vi "Test Complete.vi"(8 "Vehicle":string, 9 "SMS Recipients":u32, 10 "Send SMS":bool, 11 "File Name":string) -> ()   [LabVIEW 2014]
panel:
  out "Boolean array":bool[](array[boolean])
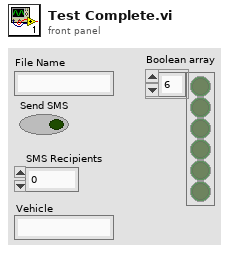
[diagram p1: front panel]
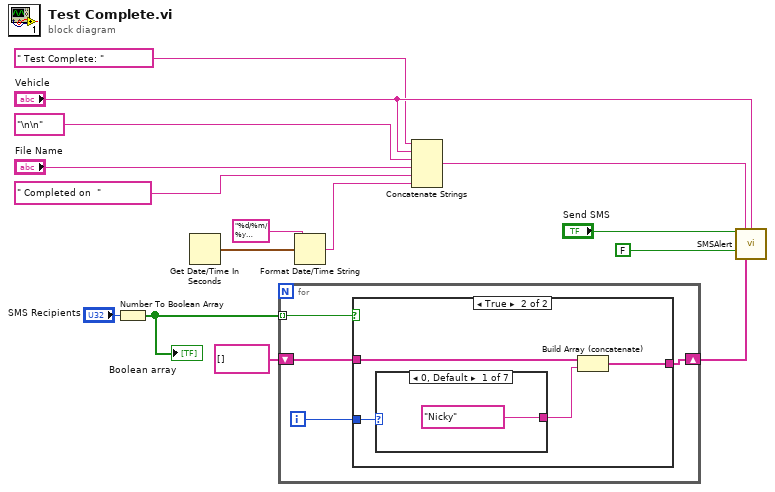
[diagram p0: block diagram]
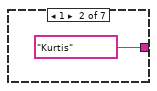
[diagram p3: hidden frame]
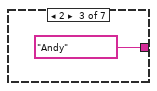
[diagram p4: hidden frame]
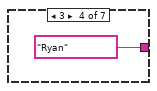
[diagram p5: hidden frame]
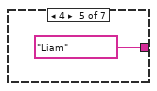
[diagram p6: hidden frame]
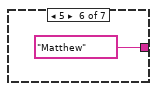
[diagram p7: hidden frame]
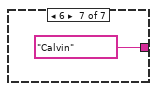
[diagram p8: hidden frame]
diagram:
  n1 = Number To Boolean Array(number="SMS Recipients") -> (Boolean array=w12:bool[])
  "Boolean array" <- w12
  n2 = Get Date/Time In Seconds() -> (seconds since 1Jan1904=w9:timestamp)
  n3 = for {
    tunnel: w12 -> [w19] mode=indexing
    shift-right: [w16] -> w10
    shift-left: string[] [] -> [w17]
    i -> [w18]
    n4 = case shown="True" w19 {
      tunnel: w18 -> [_ w24]
      tunnel: w17 -> [w20 w23]
      tunnel: [w20 w21] -> w16
      frame False {
      }
      frame True {
        n5 = case shown="0, Default" w24 {
          tunnel: ["Nicky" ("String") "Kurtis" ("String") "Andy" ("String") "Ryan" ("String") "Liam" ("String") "Matthew" ("String") "Calvin" ("String")] -> w22
          frame 0, Default {
          }
          frame 1 {
          }
          frame 2 {
          }
          frame 3 {
          }
          frame 4 {
          }
          frame 5 {
          }
          frame 6 {
          }
        }
        n6 = Build Array (concatenate)(w23, w22) -> (w21:string[])
      }
    }
  }
  n7 = Format Date/Time String(time format string (%c)="%d/%m/%y %H:%M:%S", seconds (now)=w9) -> (date/time string=w6:string)  [unwired: 1 in]
  n8 = Concatenate Strings(" Test Complete: " ("string"), "Vehicle", "\n\n" ("string"), "File Name", " Completed on  " ("string"), w6) -> (w4:string)
  n9 = call "SMSAlert.vi"("Send Message?"="Send SMS", "Error Message to be sent"=w4, "Vehicle"="Vehicle", "Error Alarm?"=FALSE, "Recipients"=w10) -> ()  [unwired: 11 in]
